vi "open excel get worksheet names.vi"(8 "error in (no error)":errorcluster, 10 "milliseconds to wait":u32, 11 "report file path":path) -> (0 "error out":errorcluster, 1 "Number of Sample Sheets":i32, 2 "worksheets count":i32, 3 "NI_report out":refnum<class "NI_report.lvclass">, 4 "start of Sample Sheets":i32, 5 "Worksheet Names":string[](array[string]))   [LabVIEW 2016]
uses:
  <vilib>/Utility/NIReport.llb/NI_report.lvclass
  <vilib>/addons/_office/NI_ReportGenerationToolkit.lvlib
  <vilib>/Utility/NIReport.llb/Excel/NI_Excel.lvclass
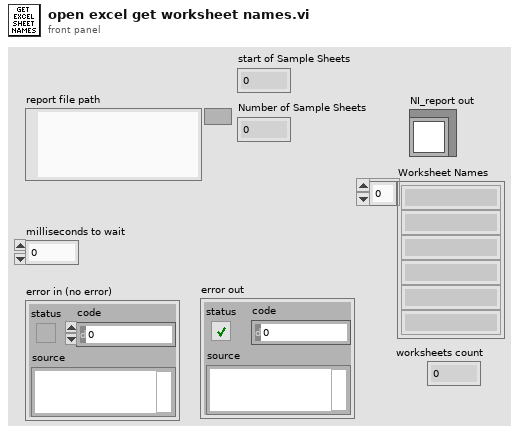
[diagram p1: front panel]
types:
  T1 = enum16{"Standard Report", "HTML", "Word", "Excel"}
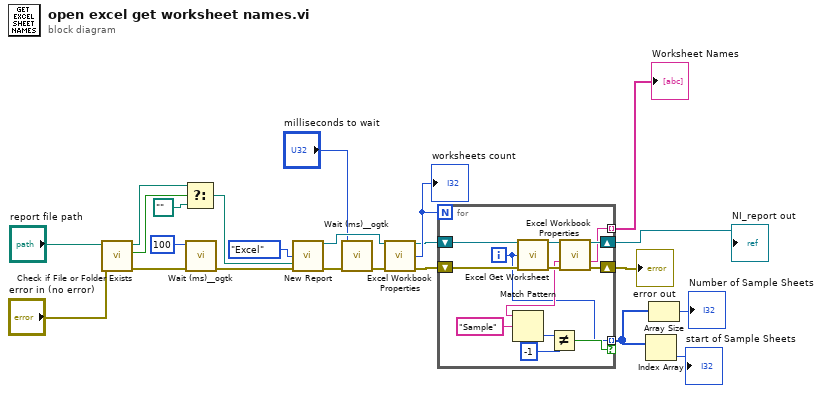
[diagram p0: block diagram]
diagram:
  n1 = call <vilib>:"Check if File or Folder Exists.vi"("error in (no error)"="error in (no error)", "path"="report file path") -> ("error out"=w7:errorcluster, "file or folder exists?"=w8:bool, "dup path"=w9:path)  [unwired: 7 in]
  n2 = Select(t=w9, s=w8, f=path "") -> (s? t:f=w10:path)
  n3 = call <userlib>:"Wait (ms)__ogtk.vi"("error in (no error)"=w7, "milliseconds to wait"=u32 100) -> ("error out"=w15:errorcluster)  [unwired: 8 in, 1 out]
  n4 = call <vilib>:"New Report.vi"("report type"=T1."Excel", "template (empty)"=w10, "error in (no error)"=w15) -> ("report out"=w17:refnum<class "NI_report.lvclass">, "error out"=w12:errorcluster)  [unwired: 11 in]
  n5 = call <userlib>:"Wait (ms)__ogtk.vi"("error in (no error)"=w12, "milliseconds to wait"="milliseconds to wait") -> ("error out"=w18:errorcluster)  [unwired: 8 in, 1 out]
  n6 = call <vilib>:"Excel Workbook Properties.vi"("report in"=w17, "error in (no error)"=w18) -> ("report out"=w20:refnum<class "NI_report.lvclass">, "worksheets count"=w21:i32, "error out"=w19:errorcluster)  [unwired: 10 in, 1 out]
  "worksheets count" <- w21
  n7 = for {
    N: w21 -> [_]
    shift-right: [w30] -> w13
    shift-left: w19 -> [w35]
    shift-right: [w31] -> w22
    shift-left: w20 -> [w34]
    tunnel: [w29] -> w23 mode=indexing
    tunnel: [w24] -> w2 mode=indexing if=w25
    i -> [w24]
    n8 = call <vilib>:"Excel Get Worksheet.vi"("report in"=w34, "worksheet index (0)"=w24, "error in (no error)"=w35) -> ("report out"=w32:refnum<class "NI_report.lvclass">, "error out"=w33:errorcluster)  [unwired: 11 in]
    n9 = call <vilib>:"Excel Workbook Properties.vi"("report in"=w32, "error in (no error)"=w33) -> ("report out"=w31:refnum<class "NI_report.lvclass">, "current worksheet name"=w29:string, "error out"=w30:errorcluster)  [unwired: 10 in, 1 out]
    n10 = Match Pattern(string=w29, regular expression="Sample") -> (offset past match=w27:i32)  [unwired: 1 in, 3 out]
    n11 = Not Equal?(x=w27, y=-1) -> (x != y?=w25:bool)
  }
  "Worksheet Names" <- w23
  "NI_report out" <- w22
  "error out" <- w13
  n12 = Index Array(array=w2) -> (element=→"start of Sample Sheets":i32)  [unwired: 1 in]
  n13 = Array Size(array=w2) -> (size(s)=→"Number of Sample Sheets":i32)
